vi "niSE Pickering Connect.vi"(8 "error in (no error)":errorcluster {"code" format="%.0x"}, 10 "Route Group(s) to Connect":string[](array[string]), 11 "Virtual Device Name":string="SwitchConfiguration1") -> (0 "error out":errorcluster)   [LabVIEW 2015]
uses:
  <vilib>/SwitchExecutive/nise.llb/niSE Expand Action Enum.ctl
panel:
  out "Routes Disconnected":string[](array[string])
  out "Routes Connected":string[](array[string])
  out "Current Connected Routes":string[](array[string])
  out "Routes to Connect":string[](array[string])
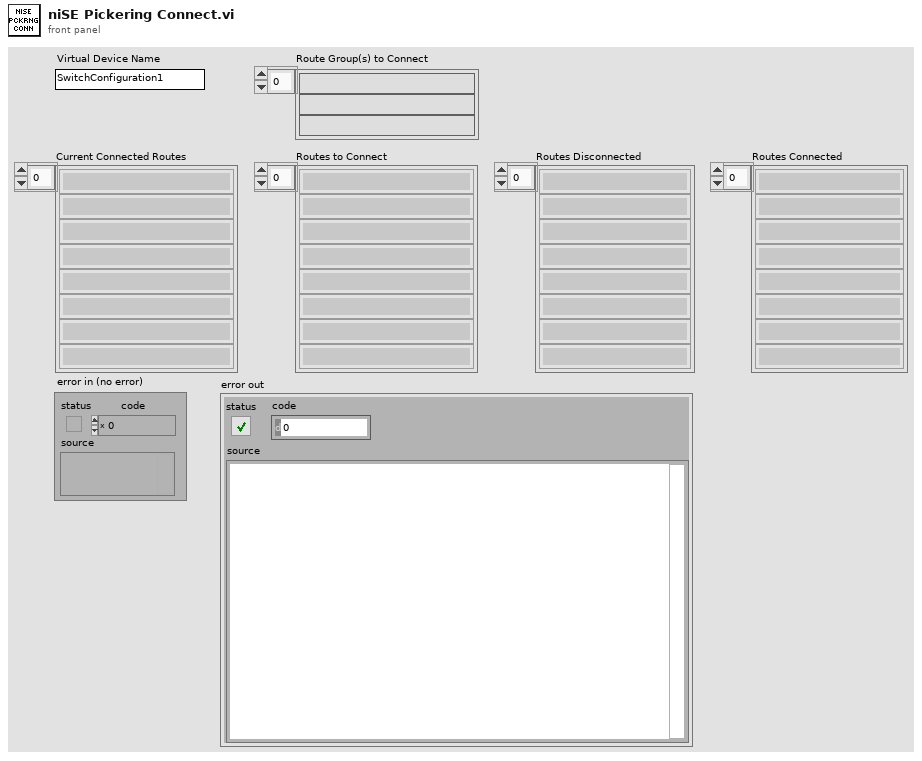
[diagram p1: front panel]
types:
  T1 = typedef "niSE Expand Action Enum.ctl" = i32
  T2 = typedef "niSE SessionRefnum.ctl" = refnum<k1>
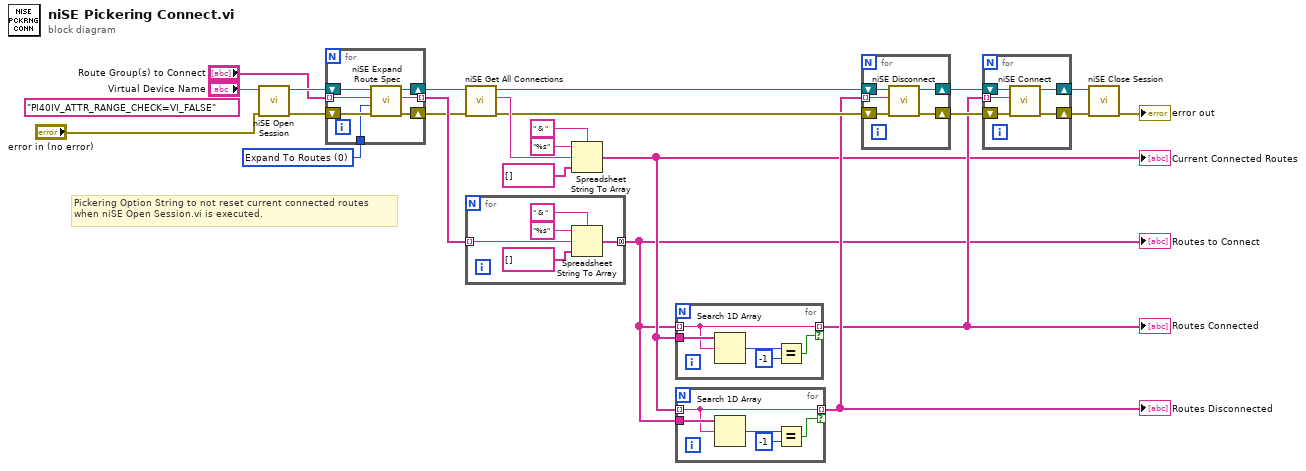
[diagram p0: block diagram]
diagram:
  (unwired) "PI40IV_ATTR_RANGE_CHECK=VI_FALSE" ("Option String (\"\")")
  w21 = T1 0 items=["Expand To Routes", "Expand To Paths"] ("Expand Action (Expand To Routes)")
  # "Pickering Option String to not reset current connected routes\nwhen niSE Open Session.vi is executed."
  n1 = call <vilib>:"niSE Open Session.vi"("error in (no error)"="error in (no error)", "Virtual Device Name (SwitchConfiguration1)"="Virtual Device Name") -> ("error out"=w23:errorcluster, "NISE Session (out)"=w22:T2)  [unwired: 4 in]
  n2 = for {
    tunnel: w21 -> [w29]
    tunnel: [w28] -> w20 mode=indexing
    tunnel: "Route Group(s) to Connect" -> [w25] mode=indexing
    shift-right: [w27] -> w19
    shift-left: w23 -> [w31]
    shift-right: [w26] -> w18
    shift-left: w22 -> [w30]
    n3 = call <vilib>:"niSE Expand Route Spec.vi"("error in (no error)"=w31, "Expand Action (Expand To Routes)"=w29, "Route Specification (\"\")"=w25, "NISE Session (in)"=w30) -> ("error out"=w27:errorcluster, "Expanded Route Specification"=w28:string, "NISE Session (out)"=w26:T2)  [unwired: 1 in]
  }
  n4 = call <vilib>:"niSE Get All Connections.vi"("error in (no error)"=w19, "NISE Session (in)"=w18) -> ("error out"=w12:errorcluster, "Route Specification"=w14:string, "NISE Session (out)"=w13:T2)  [unwired: 3 in]
  n5 = for {
    tunnel: w20 -> [w34] mode=indexing
    tunnel: [w32] -> w4 mode=concatenating
    n6 = Spreadsheet String To Array(delimiter (Tab)=" & ", format string="%s", spreadsheet string=w34, array type (2D Dbl)=string[] []) -> (array=w32:string[])
  }
  "Routes to Connect" <- w4
  n7 = Spreadsheet String To Array(delimiter (Tab)=" & ", format string="%s", spreadsheet string=w14, array type (2D Dbl)=string[] []) -> (array=w5:string[])
  "Current Connected Routes" <- w5
  n8 = for {
    tunnel: w4 -> [w38] mode=indexing
    tunnel: w5 -> [w41]
    tunnel: [w38] -> w8 mode=indexing if=w37
    n9 = Search 1D Array(1D array=w41, element=w38) -> (index of element=w40:i32)  [unwired: 1 in]
    n10 = Equal?(x=w40, y=-1) -> (x = y?=w37:bool)
  }
  "Routes Connected" <- w8
  n11 = for {
    tunnel: w5 -> [w43] mode=indexing
    tunnel: w4 -> [w46]
    tunnel: [w43] -> w11 mode=indexing if=w42
    n12 = Search 1D Array(1D array=w46, element=w43) -> (index of element=w45:i32)  [unwired: 1 in]
    n13 = Equal?(x=w45, y=-1) -> (x = y?=w42:bool)
  }
  "Routes Disconnected" <- w11
  n14 = for {
    tunnel: w11 -> [w48] mode=indexing
    shift-right: [w50] -> w10
    shift-left: w13 -> [w51]
    shift-right: [w47] -> w9
    shift-left: w12 -> [w49]
    n15 = call <vilib>:"niSE Disconnect.vi"("error in (no error)"=w49, "Disconnection Specification (\"\")"=w48, "NISE Session (in)"=w51) -> ("error out"=w47:errorcluster, "NISE Session (out)"=w50:T2)  [unwired: 3 in]
  }
  n16 = for {
    tunnel: w8 -> [w53] mode=indexing
    shift-right: [w55] -> w7
    shift-left: w10 -> [w56]
    shift-right: [w52] -> w6
    shift-left: w9 -> [w54]
    n17 = call <vilib>:"niSE Connect.vi"("error in (no error)"=w54, "Connection Specification (\"\")"=w53, "NISE Session (in)"=w56) -> ("error out"=w52:errorcluster, "NISE Session (out)"=w55:T2)  [unwired: 7 in]
  }
  n18 = call <vilib>:"niSE Close Session.vi"("error in (no error)"=w6, "NISE Session (in)"=w7) -> ("error out"=→"error out":errorcluster)  [unwired: 5 in]
